vi "SO2 TCP Packet_v2.vi"(0 "ID":string, 5 "Version":string, 7 "utc_time":u32, 9 "dummy1":string="0", 11 "dummy2":string="0", 12 "Flight Number":string, 13 "Data Array":string[](array[string])) -> (8 "TCP Binary Packet":string)   [LabVIEW 2014]
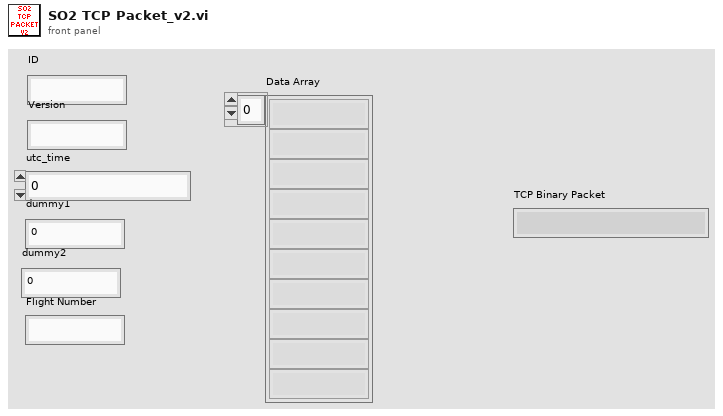
[diagram p1: front panel]
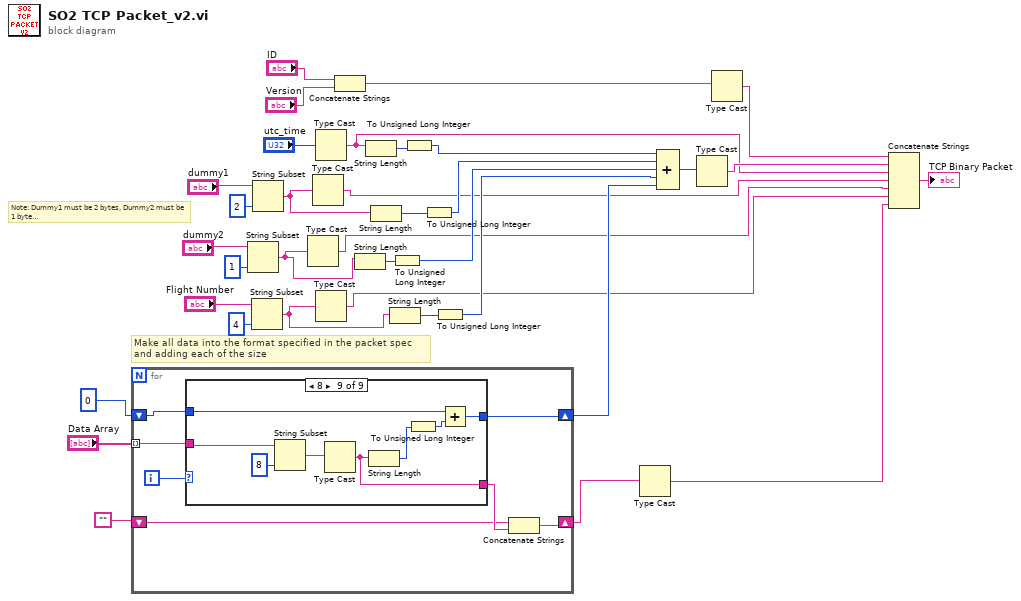
[diagram p0: block diagram]
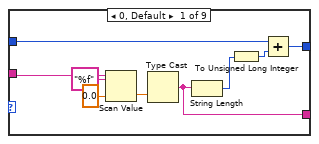
[diagram p2: hidden frame]
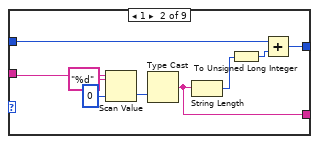
[diagram p3: hidden frame]
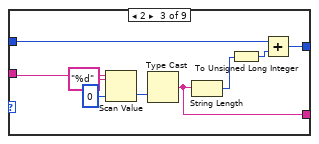
[diagram p4: hidden frame]
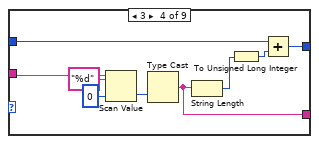
[diagram p5: hidden frame]
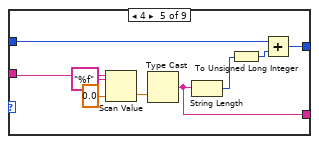
[diagram p6: hidden frame]
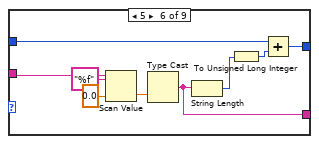
[diagram p7: hidden frame]
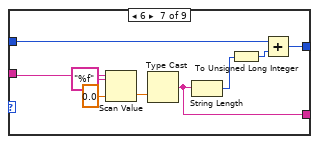
[diagram p8: hidden frame]
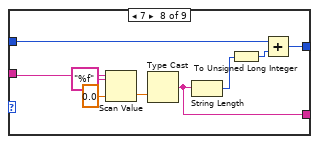
[diagram p9: hidden frame]
diagram:
  # "Note: Dummy1 must be 2 bytes, Dummy2 must be 1 byte\nin order to make the Flight number to start from byte 20"
  # "Make all data into the format specified in the packet spec\nand adding each of the size"
  n1 = for {
    tunnel: "Data Array" -> [w41] mode=indexing
    shift-right: [w39] -> w17
    shift-left: u32 0 -> [w40]
    shift-right: [w38] -> w5
    shift-left: "" -> [w36]
    i -> [w42]
    n2 = case shown="8" w42 {
      tunnel: w41 -> [w49 w58 w67 w76 w85 w94 w103 w112 w116]
      tunnel: w40 -> [w47 w56 w65 w74 w83 w92 w101 w110 w122]
      tunnel: [w44 w53 w62 w71 w80 w89 w98 w107 w119] -> w39
      tunnel: [w43 w52 w61 w70 w79 w88 w97 w106 w118] -> w37
      frame 0, Default {
        n3 = Scan Value(string=w49, format string="%f", default (0 dbl)=sgl 0.0 ("default (0 I32)")) -> (value=w51:sgl)  [unwired: 1 out]
        n4 = Type Cast(x=w51) -> (*(type *) &x=w43:string)  [unwired: 1 in]
        n5 = String Length(string=w43) -> (length=w46:i32)
        n6 = To Unsigned Long Integer(number=w46) -> (unsigned 32bit integer=w45:u32)
        n7 = Add(x=w47, y=w45) -> (x+y=w44:u32)
      }
      frame 1 {
        n8 = Scan Value(string=w58, format string="%d", default (0 dbl)=0 ("default (0 I32)")) -> (value=w60:i32)  [unwired: 1 out]
        n9 = Type Cast(x=w60) -> (*(type *) &x=w52:string)  [unwired: 1 in]
        n10 = String Length(string=w52) -> (length=w55:i32)
        n11 = To Unsigned Long Integer(number=w55) -> (unsigned 32bit integer=w54:u32)
        n12 = Add(x=w56, y=w54) -> (x+y=w53:u32)
      }
      frame 2 {
        n13 = Scan Value(string=w67, format string="%d", default (0 dbl)=0 ("default (0 I32)")) -> (value=w69:i32)  [unwired: 1 out]
        n14 = Type Cast(x=w69) -> (*(type *) &x=w61:string)  [unwired: 1 in]
        n15 = String Length(string=w61) -> (length=w64:i32)
        n16 = To Unsigned Long Integer(number=w64) -> (unsigned 32bit integer=w63:u32)
        n17 = Add(x=w65, y=w63) -> (x+y=w62:u32)
      }
      frame 3 {
        n18 = Scan Value(string=w76, format string="%d", default (0 dbl)=0 ("default (0 I32)")) -> (value=w78:i32)  [unwired: 1 out]
        n19 = Type Cast(x=w78) -> (*(type *) &x=w70:string)  [unwired: 1 in]
        n20 = String Length(string=w70) -> (length=w73:i32)
        n21 = To Unsigned Long Integer(number=w73) -> (unsigned 32bit integer=w72:u32)
        n22 = Add(x=w74, y=w72) -> (x+y=w71:u32)
      }
      frame 4 {
        n23 = Scan Value(string=w85, format string="%f", default (0 dbl)=sgl 0.0 ("default (0 I32)")) -> (value=w87:sgl)  [unwired: 1 out]
        n24 = Type Cast(x=w87) -> (*(type *) &x=w79:string)  [unwired: 1 in]
        n25 = String Length(string=w79) -> (length=w82:i32)
        n26 = To Unsigned Long Integer(number=w82) -> (unsigned 32bit integer=w81:u32)
        n27 = Add(x=w83, y=w81) -> (x+y=w80:u32)
      }
      frame 5 {
        n28 = Scan Value(string=w94, format string="%f", default (0 dbl)=sgl 0.0 ("default (0 I32)")) -> (value=w96:sgl)  [unwired: 1 out]
        n29 = Type Cast(x=w96) -> (*(type *) &x=w88:string)  [unwired: 1 in]
        n30 = String Length(string=w88) -> (length=w91:i32)
        n31 = To Unsigned Long Integer(number=w91) -> (unsigned 32bit integer=w90:u32)
        n32 = Add(x=w92, y=w90) -> (x+y=w89:u32)
      }
      frame 6 {
        n33 = Scan Value(string=w103, format string="%f", default (0 dbl)=sgl 0.0 ("default (0 I32)")) -> (value=w105:sgl)  [unwired: 1 out]
        n34 = Type Cast(x=w105) -> (*(type *) &x=w97:string)  [unwired: 1 in]
        n35 = String Length(string=w97) -> (length=w100:i32)
        n36 = To Unsigned Long Integer(number=w100) -> (unsigned 32bit integer=w99:u32)
        n37 = Add(x=w101, y=w99) -> (x+y=w98:u32)
      }
      frame 7 {
        n38 = Scan Value(string=w112, format string="%f", default (0 dbl)=sgl 0.0 ("default (0 I32)")) -> (value=w114:sgl)  [unwired: 1 out]
        n39 = Type Cast(x=w114) -> (*(type *) &x=w106:string)  [unwired: 1 in]
        n40 = String Length(string=w106) -> (length=w109:i32)
        n41 = To Unsigned Long Integer(number=w109) -> (unsigned 32bit integer=w108:u32)
        n42 = Add(x=w110, y=w108) -> (x+y=w107:u32)
      }
      frame 8 {
        n43 = String Subset(string=w116, length (rest)=8 ("length (rest)")) -> (substring=w115:string)  [unwired: 1 in]
        n44 = Type Cast(x=w115) -> (*(type *) &x=w118:string)  [unwired: 1 in]
        n45 = String Length(string=w118) -> (length=w121:i32)
        n46 = To Unsigned Long Integer(number=w121) -> (unsigned 32bit integer=w120:u32)
        n47 = Add(x=w122, y=w120) -> (x+y=w119:u32)
      }
    }
    n48 = Concatenate Strings(w36, w37) -> (w38:string)
  }
  n49 = String Subset(string="dummy2", length (rest)=1 ("length (rest)")) -> (substring=w2:string)  [unwired: 1 in]
  n50 = String Subset(string="Flight Number", length (rest)=4 ("length (rest)")) -> (substring=w9:string)  [unwired: 1 in]
  n51 = String Subset(string="dummy1", length (rest)=2 ("length (rest)")) -> (substring=w12:string)  [unwired: 1 in]
  n52 = Type Cast(x=w2) -> (*(type *) &x=w1:string)  [unwired: 1 in]
  n53 = Type Cast(x=w12) -> (*(type *) &x=w11:string)  [unwired: 1 in]
  n54 = Type Cast(x="utc_time") -> (*(type *) &x=w13:string)  [unwired: 1 in]
  n55 = Type Cast(x=w9) -> (*(type *) &x=w10:string)  [unwired: 1 in]
  n56 = Concatenate Strings("ID", "Version") -> (w33:string)
  n57 = String Length(string=w2) -> (length=w25:i32)
  n58 = String Length(string=w13) -> (length=w32:i32)
  n59 = String Length(string=w12) -> (length=w28:i32)
  n60 = String Length(string=w9) -> (length=w22:i32)
  n61 = To Unsigned Long Integer(number=w25) -> (unsigned 32bit integer=w24:u32)
  n62 = To Unsigned Long Integer(number=w32) -> (unsigned 32bit integer=w30:u32)
  n63 = To Unsigned Long Integer(number=w28) -> (unsigned 32bit integer=w26:u32)
  n64 = To Unsigned Long Integer(number=w22) -> (unsigned 32bit integer=w20:u32)
  n65 = Type Cast(x=w5) -> (*(type *) &x=w8:string)  [unwired: 1 in]
  n66 = Compound Arithmetic op=ADD(w30, w26, w24, w20, w17) -> (w15:u32)
  n67 = Type Cast(x=w15) -> (*(type *) &x=w14:string)  [unwired: 1 in]
  n68 = Type Cast(x=w33) -> (*(type *) &x=w16:string)  [unwired: 1 in]
  n69 = Concatenate Strings(w16, w14, w13, w11, w1, w10, w8) -> (→"TCP Binary Packet":string)
